vi "Joystick Control.vi"(9 "Enum":T2=enum."Run") -> (0 "Buttons Output Secondary":bool[](array[boolean]), 1 "Axis Output secondary":dbl[](array[numeric]), 2 "Button Output Primary":bool[](array[boolean]), 3 "Axis Output Primary":dbl[](array[numeric]))   [LabVIEW 2014]
uses:
  SRE Enum.ctl
  <vilib>/Rock Robotics/WPI/Joystick/WPI_JoystickDeviceEnum.ctl
panel:
  in  "Array":T1(array[ring])
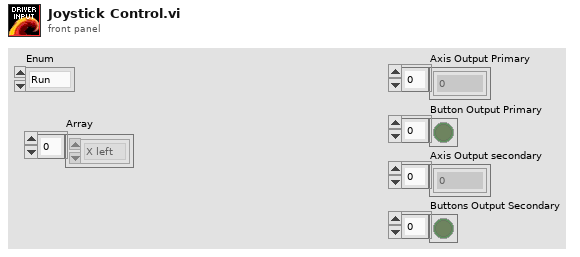
[diagram p1: front panel]
types:
  T1 = enum16{"X left ", "Y left", "Z left", "X right", "Y right", "Z right"}[]
  T2 = typedef "SRE Enum.ctl" = enum16{"Start", "Run", "End"}
  T3 = typedef "WPI_JoystickDeviceEnum.ctl" = enum16{"USB 0", "USB 1", "USB 2", "USB 3", "USB 4", "USB 5"}
  T4 = typedef "WPI_JoystickDevRef.ctl" = cluster{"Device":T3}
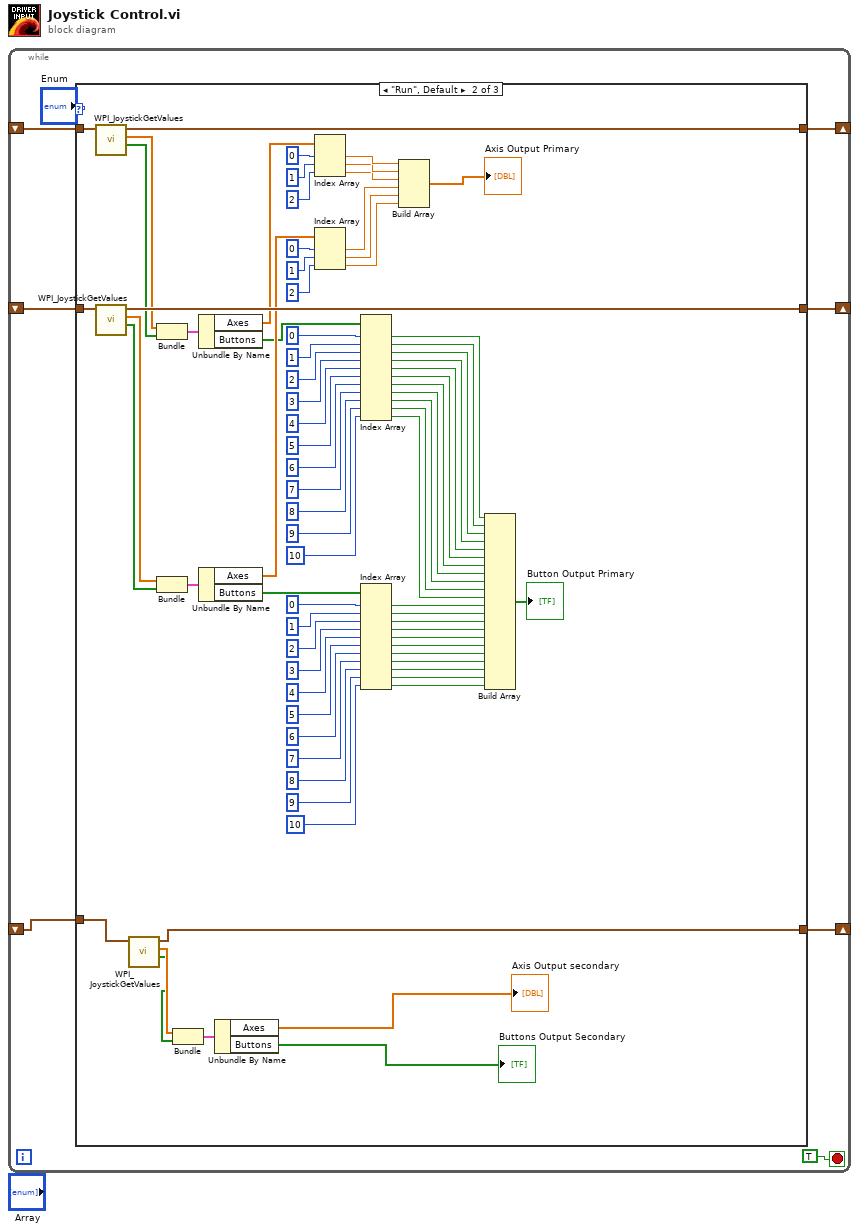
[diagram p0: block diagram]
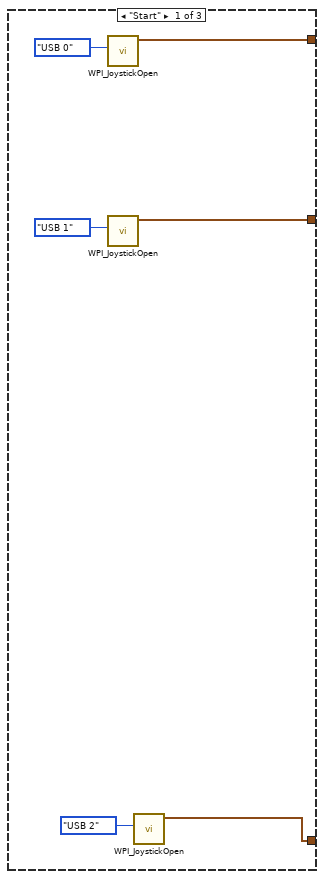
[diagram p2: hidden frame]
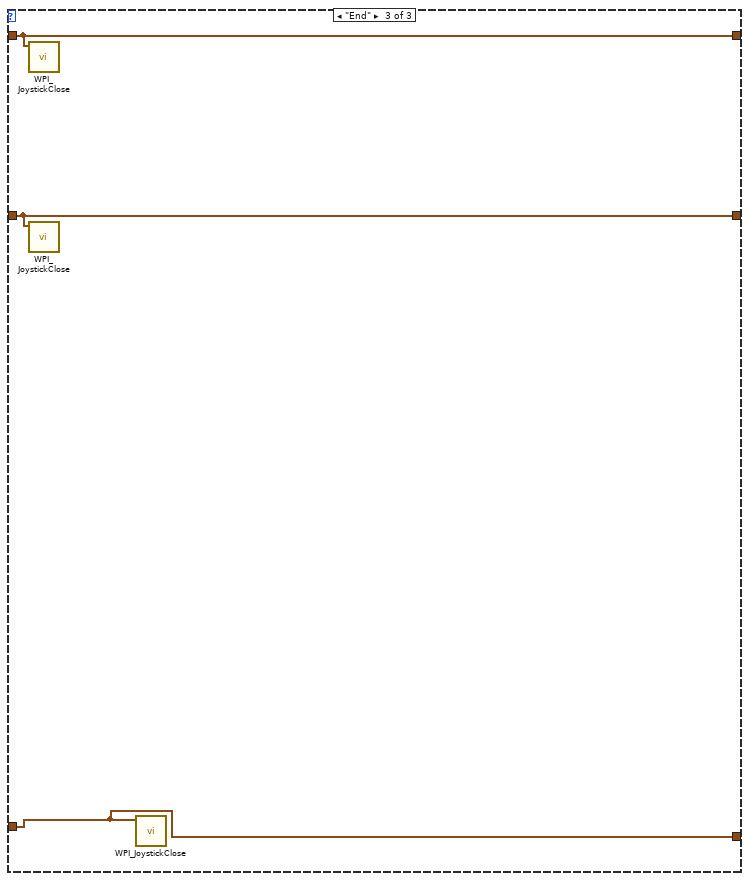
[diagram p3: hidden frame]
diagram:
  n1 = while {
    shift-right: [w7] -> _
    shift-left: _ -> [w4]
    shift-right: [w6] -> _
    shift-left: _ -> [w5]
    shift-right: [w2] -> _
    shift-left: _ -> [w1]
    stop <- TRUE stop-if-true
    n2 = case shown="\"Run\", Default" "Enum" {
      tunnel: [w14 w90 w95] -> w7
      tunnel: [w13 w92 w96] -> w6
      tunnel: w5 -> [_ w93 w96]
      tunnel: w4 -> [_ w91 w95]
      tunnel: [w9 w21 w94] -> w2
      tunnel: w1 -> [_ w20 w94]
      frame "Start" {
        n3 = call <vilib>:"WPI_JoystickOpen.vi"("JoystickDevice"=WPI_JoystickDeviceEnum."USB 0") -> ("JoystickDevRef"=w14:T4)  [unwired: 10 in]
        n4 = call <vilib>:"WPI_JoystickOpen.vi"("JoystickDevice"=WPI_JoystickDeviceEnum."USB 1") -> ("JoystickDevRef"=w13:T4)  [unwired: 10 in]
        n5 = call <vilib>:"WPI_JoystickOpen.vi"("JoystickDevice"=WPI_JoystickDeviceEnum."USB 2") -> ("JoystickDevRef"=w9:T4)  [unwired: 10 in]
      }
      frame "Run", Default {
        n6 = call <vilib>:"WPI_JoystickGetValues.vi"("JoystickDevRef"=w91) -> ("Buttons"=w88:bool[], "Axes"=w89:dbl[], "JoystickDevRef"=w90:T4)  [unwired: 6 in, 2 out]
        n7 = call <vilib>:"WPI_JoystickGetValues.vi"("JoystickDevRef"=w93) -> ("Buttons"=w86:bool[], "Axes"=w87:dbl[], "JoystickDevRef"=w92:T4)  [unwired: 6 in, 2 out]
        n8 = call <vilib>:"WPI_JoystickGetValues.vi"("JoystickDevRef"=w20) -> ("Buttons"=w17:bool[], "Axes"=w18:dbl[], "JoystickDevRef"=w21:T4)  [unwired: 6 in, 2 out]
        n9 = Bundle("Axes"=w89, "Buttons"=w88) -> (w85:cluster{"Axes":dbl[], "Buttons":bool[]})  [unwired: 1 in]
        n10 = Bundle("Axes"=w87, "Buttons"=w86) -> (w84:cluster{"Axes":dbl[], "Buttons":bool[]})  [unwired: 1 in]
        n11 = Bundle("Axes"=w18, "Buttons"=w17) -> (w19:cluster{"Axes":dbl[], "Buttons":bool[]})  [unwired: 1 in]
        n12 = Unbundle By Name(w85) -> ("Axes"=w83:dbl[], "Buttons"=w65:bool[])
        n13 = Unbundle By Name(w84) -> ("Axes"=w82:dbl[], "Buttons"=w35:bool[])
        n14 = Unbundle By Name(w19) -> ("Axes"=→"Axis Output secondary":dbl[], "Buttons"=→"Buttons Output Secondary":bool[])
        n15 = Index Array(array=w83, index #1=0 ("index"), index #2=1 ("index"), index #3=2 ("index")) -> (element #1=w75:dbl, element #2=w74:dbl, element #3=w73:dbl)
        n16 = Index Array(array=w82, index #1=0 ("index"), index #2=1 ("index"), index #3=2 ("index")) -> (element #1=w72:dbl, element #2=w71:dbl, element #3=w70:dbl)
        n17 = Index Array(array=w65, index #1=0 ("index"), index #2=1 ("index"), index #3=2 ("index"), index #4=3 ("index"), index #5=4 ("index"), index #6=5 ("index"), index #7=6 ("index"), index #8=7 ("index"), index #9=8 ("index"), index #10=9 ("index"), index #11=10 ("index")) -> (element #1=w68:bool, element #2=w67:bool, element #3=w66:bool, element #4=w52:bool, element #5=w51:bool, element #6=w50:bool, element #7=w49:bool, element #8=w48:bool, element #9=w47:bool, element #10=w46:bool, element #11=w45:bool)
        n18 = Index Array(array=w35, index #1=0 ("index"), index #2=1 ("index"), index #3=2 ("index"), index #4=3 ("index"), index #5=4 ("index"), index #6=5 ("index"), index #7=6 ("index"), index #8=7 ("index"), index #9=8 ("index"), index #10=9 ("index"), index #11=10 ("index")) -> (element #1=w32:bool, element #2=w31:bool, element #3=w30:bool, element #4=w29:bool, element #5=w28:bool, element #6=w27:bool, element #7=w26:bool, element #8=w25:bool, element #9=w24:bool, element #10=w23:bool, element #11=w22:bool)
        n19 = Build Array(w75, w74, w73, w72, w71, w70) -> (→"Axis Output Primary":dbl[])
        n20 = Build Array(w68, w67, w66, w52, w51, w50, w49, w48, w47, w46, w45, w32, w31, w30, w29, w28, w27, w26, w25, w24, w23, w22) -> (→"Button Output Primary":bool[])
      }
      frame "End" {
        n21 = call <vilib>:"WPI_JoystickClose.vi"("JoystickDevRef"=w95) -> ()  [unwired: 11 in]
        n22 = call <vilib>:"WPI_JoystickClose.vi"("JoystickDevRef"=w96) -> ()  [unwired: 11 in]
        n23 = call <vilib>:"WPI_JoystickClose.vi"("JoystickDevRef"=w94) -> ()  [unwired: 11 in]
      }
    }
  }
